vi "seq[].vi"(1 "数值":i32) -> (0 "数组":string[](array[string]))   [LabVIEW 2018]
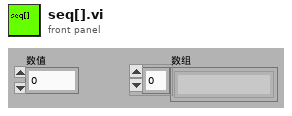
[diagram p1: front panel]
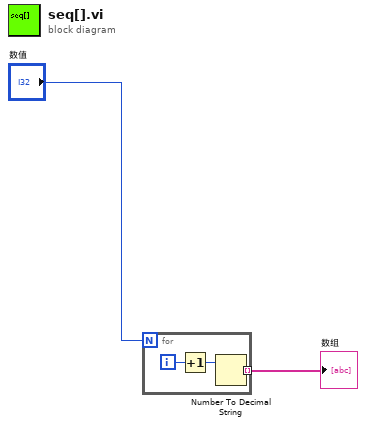
[diagram p0: block diagram]
diagram:
  n1 = for {
    N: "数值" -> [_]
    tunnel: [w3] -> w2 mode=indexing
    i -> [w5]
    n2 = Increment(x=w5) -> (x+1=w4:i32)
    n3 = Number To Decimal String(number=w4) -> (decimal integer string=w3:string)  [unwired: 1 out]
  }
  "数组" <- w2
